vi "MCList-Get Set columns size.vi"(6 "Number of columns (10)":i32=10, 7 "Function":T1, 8 "error in (no error)":errorcluster, 10 "Column Sizes":u32[](array[numeric]), 11 "Listbox ref":refnum<vi>) -> (0 "Error out":errorcluster, 2 "Sizes":u32[](array[numeric]))   [LabVIEW 2020]
uses:
  User Interface/Visualisation/Functional Imaging Viewer/Typedefs/Get-Set-Clear Control.ctl
  <vilib>/Utility/miscctls.llb/LVRowAndColumnTypeDef.ctl
panel:
  in  "Coord Listbox":i32[](listbox)
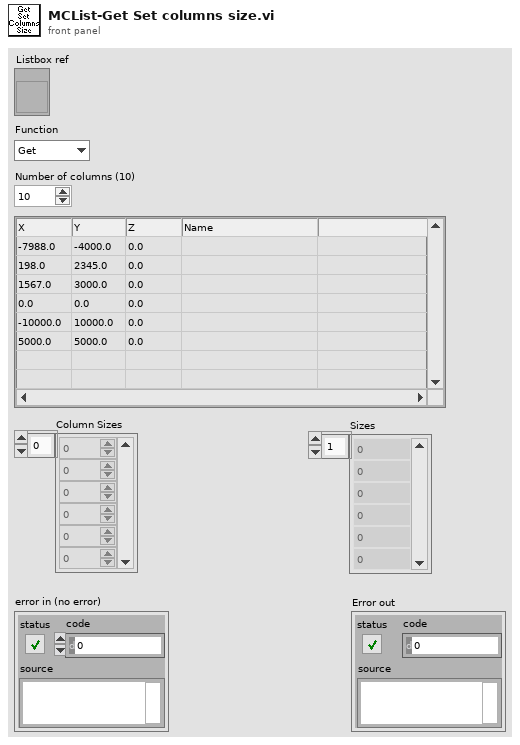
[diagram p1: front panel]
types:
  T1 = typedef "Get-Set-Clear Control.ctl" = enum16{"Get", "Set", "Clear"}
  T2 = typedef "LVRowAndColumnTypeDef.ctl" = cluster{"Row":i32, "Column":i32}
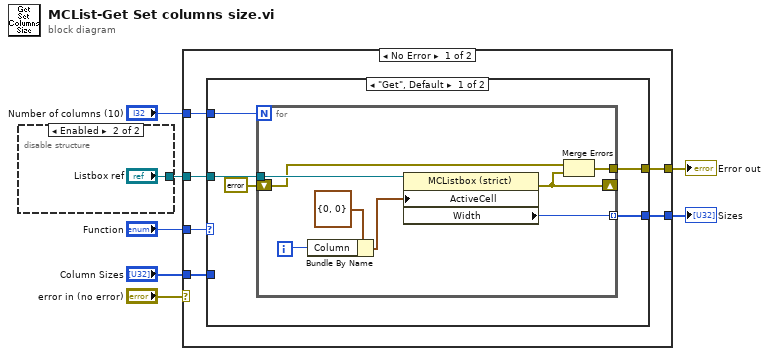
[diagram p0: block diagram]
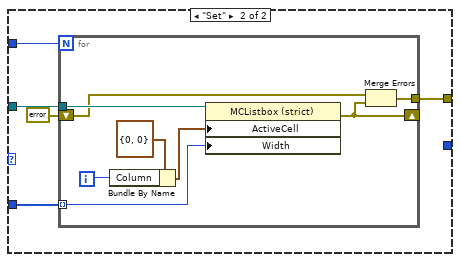
[diagram p2: hidden frame]
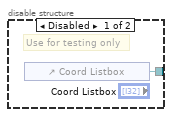
[diagram p4: hidden frame]
diagram:
  n1 = disable-structure shown="Enabled" {
    disable-tunnel: [w8 "Listbox ref"] -> w7
    frame Disabled {
      # "Use for testing only"
      n2 = control-ref of="Coord Listbox"() -> (w8:refnum<vi>)
    }
    frame Enabled {
    }
  }
  n3 = case shown="No Error" "error in (no error)" {
    selector: "error in (no error)" -> [_ w42]
    tunnel: w7 -> [w15 _]
    tunnel: [w14 w43] -> w6
    tunnel: "Number of columns (10)" -> [w13 _]
    tunnel: "Function" -> [w12 _]
    tunnel: [w11 w42] -> w3
    tunnel: "Column Sizes" -> [w10 w43]
    frame No Error {
      n4 = case shown="\"Get\", Default" w12 {
        tunnel: w15 -> [w20 w33]
        tunnel: w13 -> [w19 w32]
        tunnel: [w18 _] -> w14
        tunnel: [w16 w30] -> w11
        tunnel: w10 -> [_ w29]
        frame "Get", Default {
          n5 = for {
            N: w19 -> [_]
            tunnel: w20 -> [w28]
            tunnel: [w25] -> w18 mode=indexing
            shift-right: [w23] -> _
            shift-left: errorcluster {"status"=FALSE, "code"=0, "source"=""} ("error out") -> [w22]
            tunnel: [w21] -> w16
            i -> [w26]
            n6 = Bundle By Name(cluster=T2 {"Row"=0, "Column"=0} ("Active Cell:Active Cell"), "Column"=w26) -> (w27:T2)
            n7 = property on="Property Node" class="MCListbox (strict)"(reference=w28, "ActiveCell"=w27) -> (error out=w23:errorcluster, "Width"=w25:u32)  [unwired: 1 in, 1 out]
            n8 = Merge Errors(w22, w23) -> (w21:errorcluster)
          }
        }
        frame "Set" {
          n9 = for {
            N: w32 -> [_]
            tunnel: w33 -> [w41]
            shift-right: [w37] -> _
            shift-left: errorcluster {"status"=FALSE, "code"=0, "source"=""} ("error out") -> [w36]
            tunnel: [w35] -> w30
            tunnel: w29 -> [w34] mode=indexing
            i -> [w39]
            n10 = Bundle By Name(cluster=T2 {"Row"=0, "Column"=0} ("Active Cell:Active Cell"), "Column"=w39) -> (w40:T2)
            n11 = property on="Property Node" class="MCListbox (strict)"(reference=w41, "ActiveCell"=w40, "Width"=w34) -> (error out=w37:errorcluster)  [unwired: 1 in, 1 out]
            n12 = Merge Errors(w36, w37) -> (w35:errorcluster)
          }
        }
      }
    }
    frame Error {
    }
  }
  "Sizes" <- w6
  "Error out" <- w3
